vi "Count Numeric in TDMS Channel.vi"(6 "CHANNEL":u8, 8 "error in":errorcluster, 9 "Channel Name":string, 10 "Group Name":string, 11 "Refnum in":refnum<k34>) -> (0 "error out":errorcluster, 1 "Count":i32, 2 "group name out":string, 3 "Refnum out":refnum<k34>)   [LabVIEW 2023]
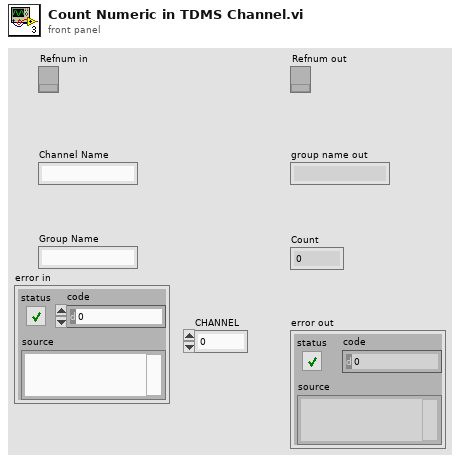
[diagram p1: front panel]
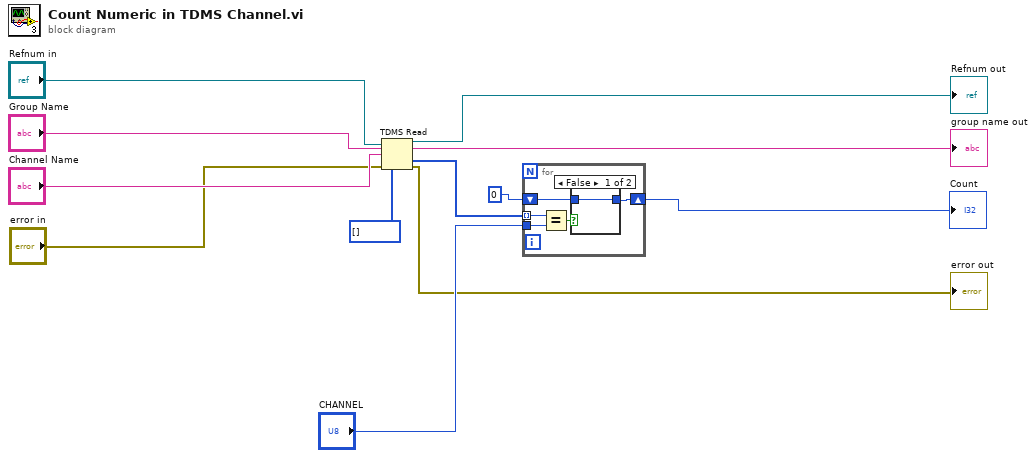
[diagram p0: block diagram]
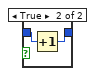
[diagram p2: hidden frame]
diagram:
  n1 = TDMS Read(0:"Refnum in", 5:"Group Name", 7:"Channel Name", 11:"error in", 12:i32[] []) -> (4:→"Refnum out":refnum<k34>, 6:→"group name out":string, 10:w11:i32[], 15:→"error out":errorcluster)  [unwired: 3 in, 2 out]
  n2 = for {
    tunnel: "CHANNEL" -> [w17]
    tunnel: w11 -> [w16] mode=indexing
    shift-right: [w13] -> w1
    shift-left: 0 -> [w14]
    n3 = Equal?(x=w16, y=w17) -> (x = y?=w15:bool)
    n4 = case shown="False" w15 {
      tunnel: w14 -> [w18 w20]
      tunnel: [w18 w19] -> w13
      frame False {
      }
      frame True {
        n5 = Increment(x=w20) -> (x+1=w19:i32)
      }
    }
  }
  "Count" <- w1
